vi "VCS Get Baudrate Selection.vi"(8 "error in (no error)":errorcluster, 10 "startOfSelection":i32, 11 "device in":T1={"deviceName"="EPOS2", "protocolStackName"="MAXON SERIAL V2", "interfaceName"="USB", "portName"="USB0"}) -> (0 "error out":errorcluster, 1 "baudrateSel":u32, 2 "endOfSelection":i32, 3 "device out":T1={"deviceName"="EPOS2", "protocolStackName"="", "interfaceName"="", "portName"=""})   [LabVIEW 2017, in "maxonEPOS.lvlib"]
doc: "VI <B>VCS Get Baudrate Selection</B> returns all available baud rates for the connected port."
uses:
  Examples/maxonEPOS.lvlib
  SSI_Tool/InstrumentsInterfaces/Motordriver/maxon EPOS/Resources/EposCmd.dll
  SSI_Tool/InstrumentsInterfaces/Motordriver/maxon EPOS/Resources/EposCmd64.dll
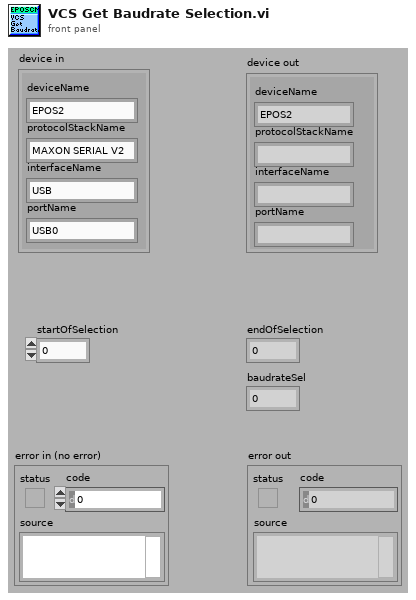
[diagram p1: front panel]
types:
  T1 = cluster{"deviceName":string, "protocolStackName":string, "interfaceName":string, "portName":string}
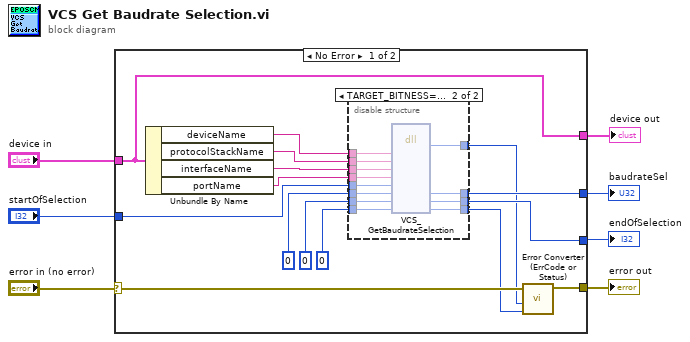
[diagram p0: block diagram]
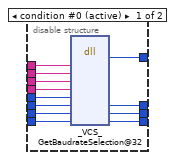
[diagram p2: hidden frame]
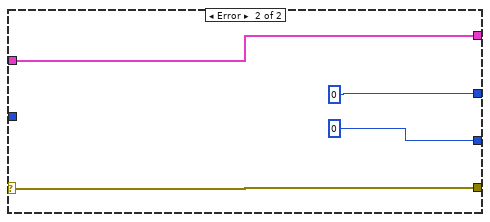
[diagram p3: hidden frame]
diagram:
  n1 = case shown="No Error" "error in (no error)" {
    selector: "error in (no error)" -> [w19 w50]
    tunnel: [w18 w50] -> w6
    tunnel: "startOfSelection" -> [w22 _]
    tunnel: [w21 u32 0 ("BaudrateSel")] -> w4
    tunnel: [w20 0 ("pEndOfSelection")] -> w3
    tunnel: "device in" -> [w9 w49]
    tunnel: [w9 w49] -> w1
    frame No Error {
      n2 = Unbundle By Name(w9) -> ("deviceName"=w16:string, "protocolStackName"=w15:string, "interfaceName"=w14:string, "portName"=w13:string)
      n3 = disable-structure shown="TARGET_BITNESS==64" {
        disable-tunnel: w22 -> [w34 w43]
        disable-tunnel: [w33 w35] -> w21
        disable-tunnel: [w32 w36] -> w20
        disable-tunnel: [w31 w37] -> w17
        disable-tunnel: w16 -> [w30 w46]
        disable-tunnel: w15 -> [w29 w45]
        disable-tunnel: w14 -> [w28 w39]
        disable-tunnel: w13 -> [w27 w44]
        disable-tunnel: u32 0 ("BaudrateSel") -> [w26 w42]
        disable-tunnel: 0 ("pEndOfSelection") -> [w25 w41]
        disable-tunnel: u32 0 ("pErrorCode") -> [w24 w40]
        disable-tunnel: [w23 w38] -> w8
        frame condition #0 (active) {
          n4 = dll-call lib="C:/workspace/project/scancon/sw/SSI_Tool/InstrumentsInterfaces/Motordriver/maxon EPOS/Resources/EposCmd.*" fn="_VCS_GetBaudrateSelection@32"("DeviceName"=w30, "ProtocolStackName"=w29, "InterfaceName"=w28, "PortName"=w27, "StartOfSelection"=w34, "BaudrateSel"=w26, "pEndOfSelection"=w25, "pErrorCode"=w24) -> (w23:i32, "BaudrateSel"=w33:u32, "pEndOfSelection"=w32:i32, "pErrorCode"=w31:u32)  [unwired: 8 in, 2 out]
        }
        frame condition #1 {
          n5 = dll-call lib="C:/setup/Resources/EposCmd64.dll" fn="VCS_GetBaudrateSelection" ("EposCmd.dll:_VCS_GetBaudrateSelection@32")("DeviceName"=w46, "ProtocolStackName"=w45, "InterfaceName"=w39, "PortName"=w44, "StartOfSelection"=w43, "BaudrateSel"=w42, "pEndOfSelection"=w41, "pErrorCode"=w40) -> ("Rückgabetyp"=w38:i32, "BaudrateSel"=w35:u32, "pEndOfSelection"=w36:i32, "pErrorCode"=w37:u32)  [unwired: 8 in, 2 out]
        }
      }
      n6 = call "Error Converter (ErrCode or Status).vi"("error code"=w17, "return type"=w8, "error in (no error)"=w19) -> ("error out"=w18:errorcluster)  [unwired: 7 in]
    }
    frame Error {
    }
  }
  "baudrateSel" <- w4
  "endOfSelection" <- w3
  "error out" <- w6
  "device out" <- w1
